vi "JoyStickPackager.vi"(9 "Buttons":bool[](array[boolean]), 10 "Axes":dbl[](array[numeric])) -> (2 "JoyStick":T1)   [LabVIEW 2018]
uses:
  Typedefs/typedef_cluster_Joystick.ctl
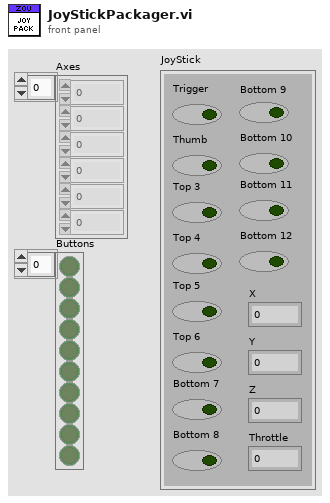
[diagram p1: front panel]
types:
  T1 = typedef "typedef_cluster_Joystick.ctl" = cluster{"X":dbl, "Y":dbl, "Z":dbl, "Throttle":dbl, "Trigger":bool, "Thumb":bool, "Top 3":bool, "Top 4":bool, "Top 5":bool, "Top 6":bool, "Bottom 7":bool, "Bottom 8":bool, "Bottom 9":bool, "Bottom 10":bool, "Bottom 11":bool, "Bottom 12":bool}
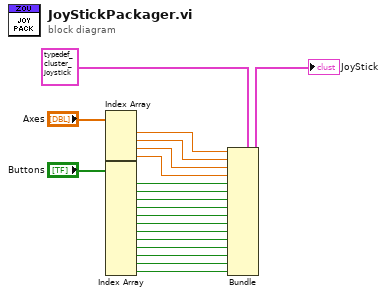
[diagram p0: block diagram]
diagram:
  n1 = Index Array(array="Axes") -> (element #1=w20:dbl, element #2=w16:dbl, element #3=w15:dbl, element #4=w14:dbl)  [unwired: 4 in]
  n2 = Index Array(array="Buttons") -> (element #1=w13:bool, element #2=w12:bool, element #3=w11:bool, element #4=w10:bool, element #5=w9:bool, element #6=w8:bool, element #7=w7:bool, element #8=w6:bool, element #9=w5:bool, element #10=w4:bool, element #11=w3:bool, element #12=w2:bool)  [unwired: 12 in]
  n3 = Bundle(cluster=T1 {"X"=0.0, "Y"=0.0, "Z"=0.0, "Throttle"=0.0, "Trigger"=FALSE, "Thumb"=FALSE, "Top 3"=FALSE, "Top 4"=FALSE, "Top 5"=FALSE, "Top 6"=FALSE, "Bottom 7"=FALSE, "Bottom 8"=FALSE, "Bottom 9"=FALSE, "Bottom 10"=FALSE, "Bottom 11"=FALSE, "Bottom 12"=FALSE} ("JoyStick"), "X"=w20, "Y"=w16, "Z"=w15, "Throttle"=w14, "Trigger"=w13, "Thumb"=w12, "Top 3"=w11, "Top 4"=w10, "Top 5"=w9, "Top 6"=w8, "Bottom 7"=w7, "Bottom 8"=w6, "Bottom 9"=w5, "Bottom 10"=w4, "Bottom 11"=w3, "Bottom 12"=w2) -> (→"JoyStick":T1)
